vi "Initialize AI Instrument.vi"(0 "DAQNode Dict":T1, 2 "offsets":T2, 5 "AI Channels":T3[](array[typedef]) {"Force Bridge"."scaling information"."physical units" items=["Newtons"=15875, "Pounds"=15876, "kgf"=15877]; "Force Bridge"."scaling information"."electrical units" items=["Volts/Volt"=15896, "mVolts/Volt"=15897]; "Force Bridge"."bridge information"."voltage excitation source" items=["Internal"=10200, "External"=10167]; "Force Bridge"."bridge information"."bridge configuration" items=["Full Bridge"=10182, "Half Bridge"=10187, "Quarter Bridge"=10270]; "Conversion"."ScaleOffset" format="%.3f"; "Conversion"."MinEngUnit" format="%.3f"; "Conversion"."MaxEngUnit" format="%.3f"; "Conversion"."MinSignal" format="%.3f"; "Conversion"."MaxSignal" format="%.3f"; "Terminal Configuration" items=["default"=-1, "RSE"=10083, "NRSE"=10078, "Differential"=10106, "Pseudodifferential"=12529]}, 7 "AI TaskName":string, 9 "Simulate":bool, 11 "error in (no error)":errorcluster) -> (4 "DAQNode Dict out":T1, 6 "AI IONames":string[](array[string]), 8 "AI SchemNames":string[](array[string]), 10 "DAQmx Task AI":refnum<k21>, 15 "error out":errorcluster)   [LabVIEW 2017, in "DAQ.lvclass"]
doc: "Developed by Kevin Thompson\nkevin@thompsonengineering.net\n\nCopyright 2018-2020\nThompson Engineering, LLC"
uses:
  DAQ.lvclass
  DataTypes/TD AI Channel--cluster.ctl
  DataTypes/TD DataValueConversion--cluster.ctl
  DataTypes/TD AI DAQ Type--enum.ctl
  DataTypes/TD AI Force Bridge--cluster.ctl
  <vilib>/TELLC/Dynamic CVT API/TD Dynamic CVT DVR--ref.ctl
  DataTypes/offsets cluster.ctl
  DataTypes/TD AI TaskIO.ctl
  <vilib>/DAQmx/create/channels.llb/DAQmx Create Channel (AI-Voltage-Basic).vi
  <vilib>/DAQmx/create/channels.llb/DAQmx Create Channel (AI-Strain-Strain Gage).vi
  <vilib>/DAQmx/create/channels.llb/DAQmx Create Channel (AI-Force-Bridge-Two-Point-Linear).vi
  <vilib>/DAQmx/create/channels.llb/DAQmx Create Channel (AI-Current-Basic).vi
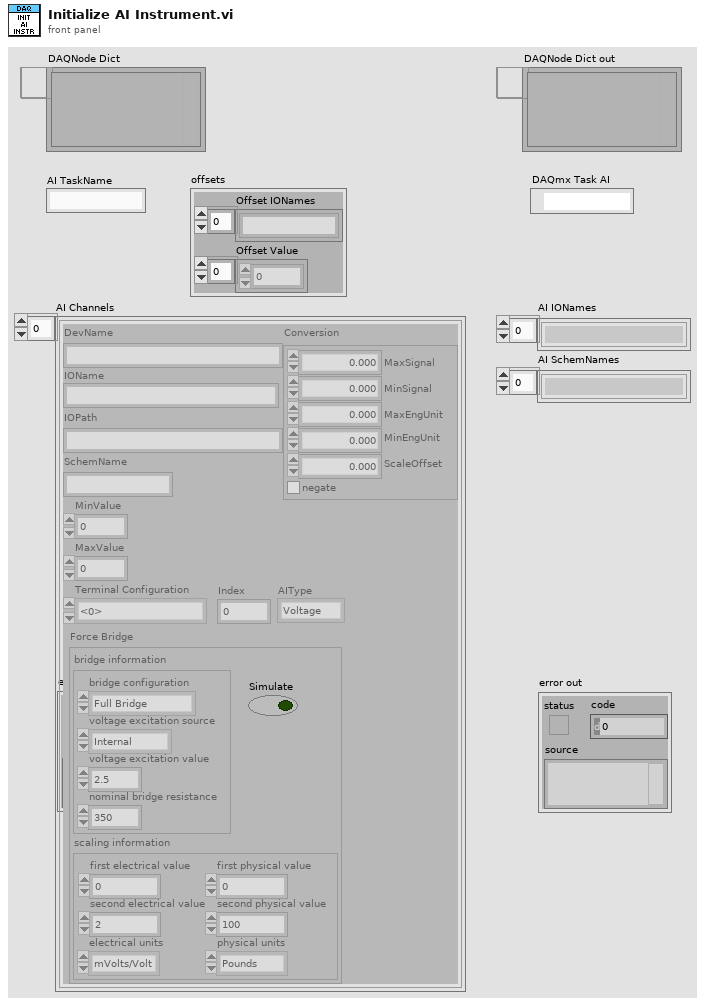
[diagram p1: front panel]
types:
  T1 = typedef "TD Dynamic CVT DVR--ref.ctl" = refnum<data-value>
  T2 = typedef "DAQ.lvclass/offsets cluster.ctl" = cluster{"Offset IONames":string[], "Offset Value":dbl[]}
  T3 = typedef "DAQ.lvclass/TD AI Channel--cluster.ctl" = cluster{"DevName":string, "IOName":string, "IOPath":string, "SchemName":string, "MinValue":dbl, "MaxValue":dbl, "Terminal Configuration":i32, "Index":i32, "Conversion":T4, "AIType":T5, "Force Bridge":T6}
  T4 = typedef "DAQ.lvclass/TD DataValueConversion--cluster.ctl" = cluster{"MaxSignal":dbl, "MinSignal":dbl, "MaxEngUnit":dbl, "MinEngUnit":dbl, "ScaleOffset":dbl, "negate":bool}
  T5 = typedef "DAQ.lvclass/TD AI DAQ Type--enum.ctl" = enum16{"Voltage", "Current", "Strain Gage", "Force Bridge"}
  T6 = typedef "DAQ.lvclass/TD AI Force Bridge--cluster.ctl" = cluster{"bridge information":cluster{"bridge configuration":i32, "voltage excitation source":i32, "voltage excitation value":dbl, "nominal bridge resistance":dbl}, "scaling information":cluster{"first electrical value":dbl, "second electrical value":dbl, "electrical units":i32, "first physical value":dbl, "second physical value":dbl, "physical units":i32}}
  T7 = typedef "DAQ.lvclass/TD AI TaskIO.ctl" = cluster{"AI TaskName":string, "IONames":string[], "DAQmx AI TaskRef":refnum<k21>}
  T8 = cluster{"bridge configuration":i32, "voltage excitation source":i32, "voltage excitation value":dbl, "nominal bridge resistance":dbl}
  T9 = cluster{"first electrical value":dbl, "second electrical value":dbl, "electrical units":i32, "first physical value":dbl, "second physical value":dbl, "physical units":i32}
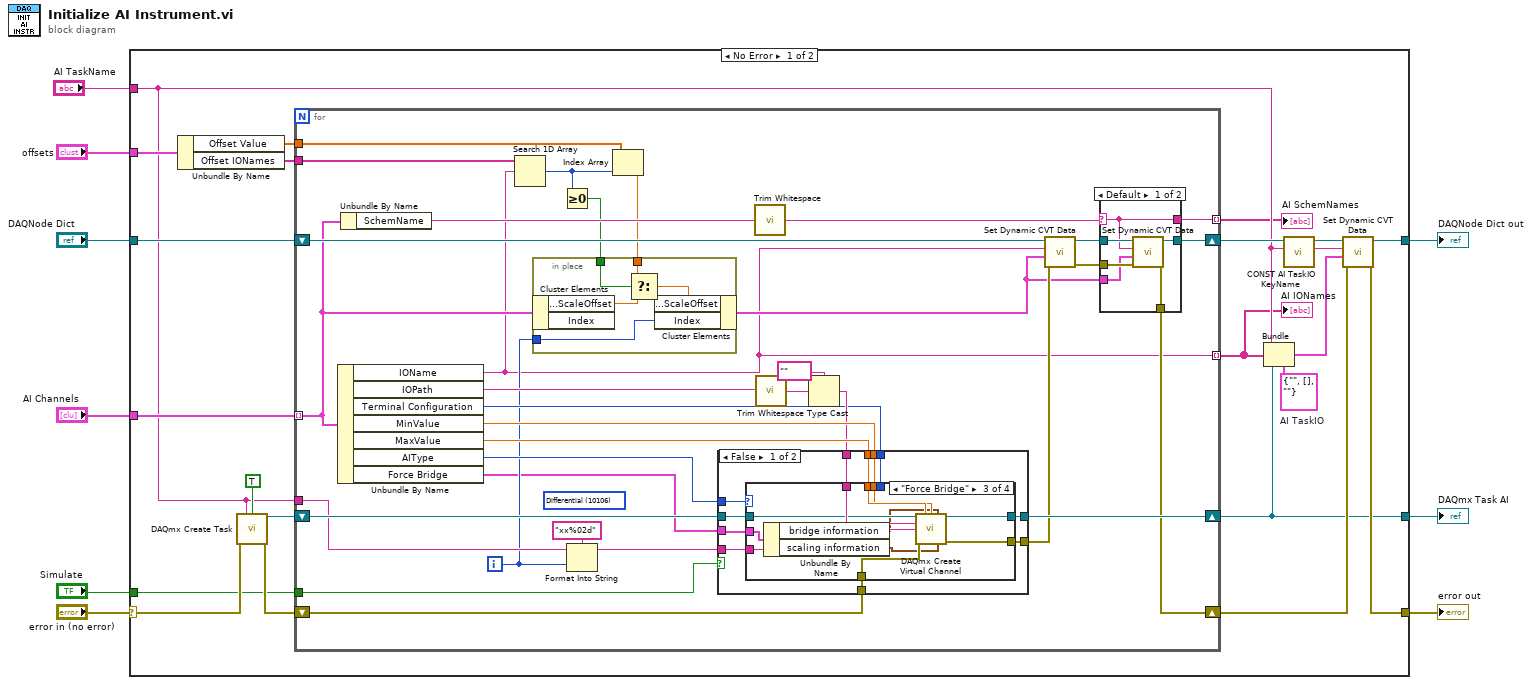
[diagram p0: block diagram]
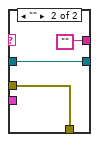
[diagram p2: hidden frame]
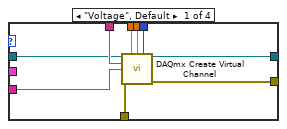
[diagram p3: hidden frame]
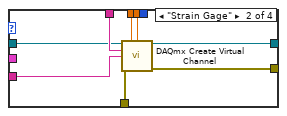
[diagram p4: hidden frame]
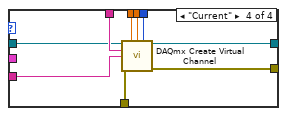
[diagram p5: hidden frame]
diagram:
  n1 = case shown="No Error" "error in (no error)" {
    selector: "error in (no error)" -> [w26 w130]
    tunnel: [w17 w130] -> w8
    tunnel: "AI Channels" -> [w27 _]
    tunnel: "Simulate" -> [w25 _]
    tunnel: "DAQNode Dict" -> [w24 w129]
    tunnel: "offsets" -> [w23 _]
    tunnel: [w19 w129] -> w3
    tunnel: [w13 _] -> w2
    tunnel: "AI TaskName" -> [w14 _]
    frame No Error {
      w12 = T7 {"AI TaskName"="", "IONames"=[], "DAQmx AI TaskRef"=""}  # AI TaskIO
      n2 = Unbundle By Name(w23) -> ("Offset Value"=w21:dbl[], "Offset IONames"=w22:string[])
      n3 = call <vilib>:"DAQmx Create Task.vi"("new task name"=w14, "auto cleanup"=TRUE, "error in"=w26) -> ("task out"=w30:refnum<k21>, "error out"=w29:errorcluster)  [unwired: 11 in]
      n4 = for {
        tunnel: w27 -> [w45] mode=indexing
        shift-right: [w50] -> w18
        shift-left: w29 -> [w54]
        shift-right: [w52] -> w20
        shift-left: w24 -> [w57]
        shift-right: [w55] -> w13
        shift-left: w30 -> [w56]
        tunnel: w14 -> [w41]
        tunnel: w25 -> [w40]
        tunnel: w22 -> [w35]
        tunnel: w21 -> [w39]
        tunnel: [w36] -> w10 mode=indexing
        tunnel: [w32] -> w11 mode=indexing
        i -> [w37]
        (unwired) 10106 items=["Default"=-1, "RSE"=10083, "NRSE"=10078, "Differential"=10106, "Pseudodifferential"=12529] ("input terminal configuration")
        n5 = Unbundle By Name(w45) -> ("IOName"=w36:string, "IOPath"=w61:string, "Terminal Configuration"=w43:i32, "MinValue"=w63:dbl, "MaxValue"=w64:dbl, "AIType"=w38:T5, "Force Bridge"=w31:T6)
        n6 = Unbundle By Name(w45) -> ("SchemName"=w49:string)
        n7 = Search 1D Array(1D array=w35, element=w36) -> (index of element=w34:i32)  [unwired: 1 in]
        n8 = Greater Or Equal To 0?(x=w34) -> (x >= 0?=w33:bool)
        n9 = Format Into String(format string="xx%02d", initial string=w41, w37) -> (resulting string=w58:string)  [unwired: 1 in, 1 out]
        n10 = Index Array(array=w39, index=w34) -> (element=w42:dbl)
        n11 = in-place {
          in-place-border: w37 -> [w69]
          in-place-border: w42 -> [w68]
          in-place-border: w33 -> [w67]
          n12 = in-place-cluster #1(w45) -> ("Conversion.ScaleOffset"=w65:dbl)  [unwired: 1 out]
          n13 = Select(t=w68, s=w67, f=w65) -> (s? t:f=w66:dbl)
          n14 = in-place-cluster #1("Conversion.ScaleOffset"=w66, "Index"=w69) -> (w44:T3)
        }
        n15 = call <vilib>:"Trim Whitespace.vi"("string"=w49) -> ("trimmed string"=w47:string)  [unwired: 1 in]
        n16 = call <vilib>:"Trim Whitespace.vi"("string"=w61) -> ("trimmed string"=w48:string)  [unwired: 1 in]
        n17 = Type Cast(type=tag "" ("physical channels"), x=w48) -> (*(type *) &x=w60:tag)
        n18 = case shown="False" w40 {
          tunnel: w64 -> [w89 _]
          tunnel: w63 -> [w88 _]
          tunnel: w60 -> [w87 _]
          tunnel: w58 -> [w86 _]
          tunnel: w56 -> [w85 w128]
          tunnel: [w84 w128] -> w55
          tunnel: w54 -> [w83 w127]
          tunnel: w43 -> [w82 _]
          tunnel: [w81 w127] -> w46
          tunnel: w38 -> [w80 _]
          tunnel: w31 -> [w79 _]
          frame False {
            n19 = case shown="\"Force Bridge\"" w80 {
              tunnel: w89 -> [w98 w106 w117 w126]
              tunnel: w88 -> [w97 w105 w116 w125]
              tunnel: w87 -> [w96 w104 w115 w124]
              tunnel: w86 -> [w95 w103 w114 w123]
              tunnel: w85 -> [w94 w102 w113 w122]
              tunnel: [w93 w101 w112 w121] -> w84
              tunnel: w83 -> [w92 w100 w111 w120]
              tunnel: w82 -> [w91 _ _ w119]
              tunnel: [w90 w99 w110 w118] -> w81
              tunnel: w79 -> [_ _ w109 _]
              frame "Voltage", Default {
                n20 = call-poly <vilib>:"DAQmx Create Virtual Channel.vi"("task in"=w94, "maximum value"=w98, "minimum value"=w97, "input terminal configuration"=w91, "physical channels"=w96, "name to assign"=w95, "error in"=w92) -> ("task out"=w93:refnum<k21>, "error out"=w90:errorcluster)  [unwired: 7 in]
              }
              frame "Strain Gage" {
                n21 = call-poly <vilib>:"DAQmx Create Virtual Channel.vi"("task in"=w102, "maximum value"=w106, "minimum value"=w105, "physical channels"=w104, "name to assign"=w103, "error in"=w100) -> ("task out"=w101:refnum<k21>, "error out"=w99:errorcluster)  [unwired: 8 in]
              }
              frame "Force Bridge" {
                n22 = Unbundle By Name(w109) -> ("bridge information"=w108:T8, "scaling information"=w107:T9)
                n23 = call-poly <vilib>:"DAQmx Create Virtual Channel.vi"("task in"=w113, "maximum value"=w117, "minimum value"=w116, "bridge information"=w108, "physical channels"=w115, "name to assign"=w114, "error in"=w111, "scaling information"=w107) -> ("task out"=w112:refnum<k21>, "error out"=w110:errorcluster)  [unwired: 6 in]
              }
              frame "Current" {
                n24 = call-poly <vilib>:"DAQmx Create Virtual Channel.vi"("task in"=w122, "maximum value"=w126, "minimum value"=w125, "input terminal configuration"=w119, "physical channels"=w124, "name to assign"=w123, "error in"=w120) -> ("task out"=w121:refnum<k21>, "error out"=w118:errorcluster)  [unwired: 7 in]
              }
            }
          }
          frame True {
          }
        }
        n25 = call <vilib>:"Set Dynamic CVT Data.vi"("error in (no error)"=w46, "value"=w44, "DataName"=w36, "dCVT DVR"=w57) -> ("error out"=w51:errorcluster, "dCVT DVR out"=w53:T1)  [unwired: 5 in, 1 out]
        n26 = case shown="Default" w47 {
          selector: w47 -> [w70 _]
          tunnel: w53 -> [w75 w77]
          tunnel: [w74 w77] -> w52
          tunnel: w51 -> [w73 w78]
          tunnel: [w72 w78] -> w50
          tunnel: w44 -> [w71 _]
          tunnel: [w70 ""] -> w32
          frame Default {
            n27 = call <vilib>:"Set Dynamic CVT Data.vi"("error in (no error)"=w73, "value"=w71, "DataName"=w70, "dCVT DVR"=w75) -> ("error out"=w72:errorcluster, "dCVT DVR out"=w74:T1)  [unwired: 5 in, 1 out]
          }
          frame "" {
          }
        }
      }
      "AI SchemNames" <- w11
      "AI IONames" <- w10
      n28 = Bundle(cluster=w12, "AI TaskName"=w14, "IONames"=w10, "DAQmx AI TaskRef"=w13) -> (w16:T7)
      n29 = call "CONST AI TaskIO KeyName.vi"("AI TaskName"=w14) -> ("AI TaskIO (KeyName)"=w15:string)  [unwired: 10 in]
      n30 = call <vilib>:"Set Dynamic CVT Data.vi"("error in (no error)"=w18, "value"=w16, "DataName"=w15, "dCVT DVR"=w20) -> ("error out"=w17:errorcluster, "dCVT DVR out"=w19:T1)  [unwired: 5 in, 1 out]
    }
    frame Error {
    }
  }
  "error out" <- w8
  "DAQNode Dict out" <- w3
  "DAQmx Task AI" <- w2
